vi "Read_Selected_channels.vi"(0 "Filename":path, 1 "Valid Channel Options":string[][](array[string]), 2 "Template Names":string[](array[string]), 3 "Data string":string, 5 "All Channels Present":string[](array[string]), 6 "End Of File already Reached?":bool, 9 "Start of data (bytes)":i32, 12 "Filetype":string, 14 "Ignore When":string[][](array[string])) -> (4 "Non-Blank Rows":i32[](array[numeric]), 8 "Deleted Rows":string[][](array[string]), 10 "Output Values":string[][](array[string]))   [LabVIEW 2015]
uses:
  Data_plotting_vis/Results_plotter_Global.vi
panel:
  out "Case":string
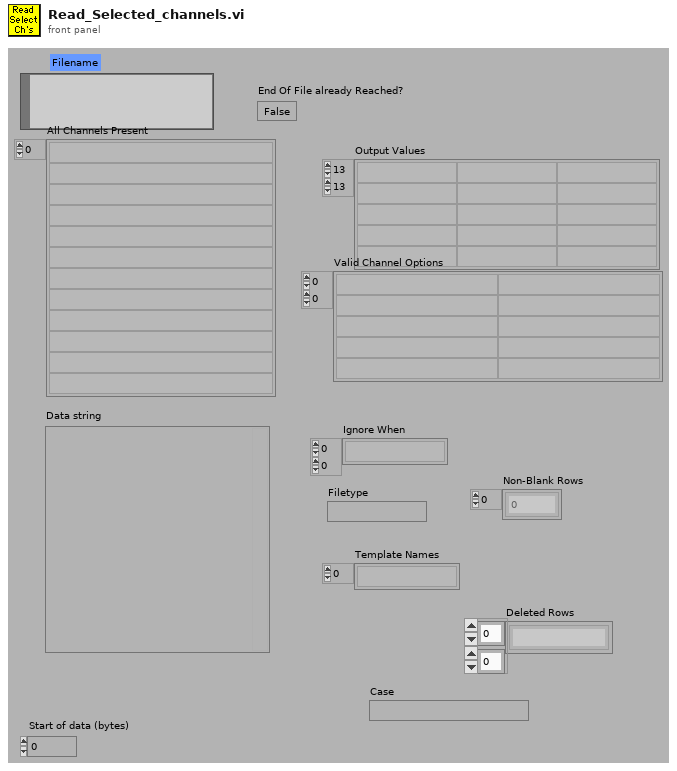
[diagram p1: front panel]
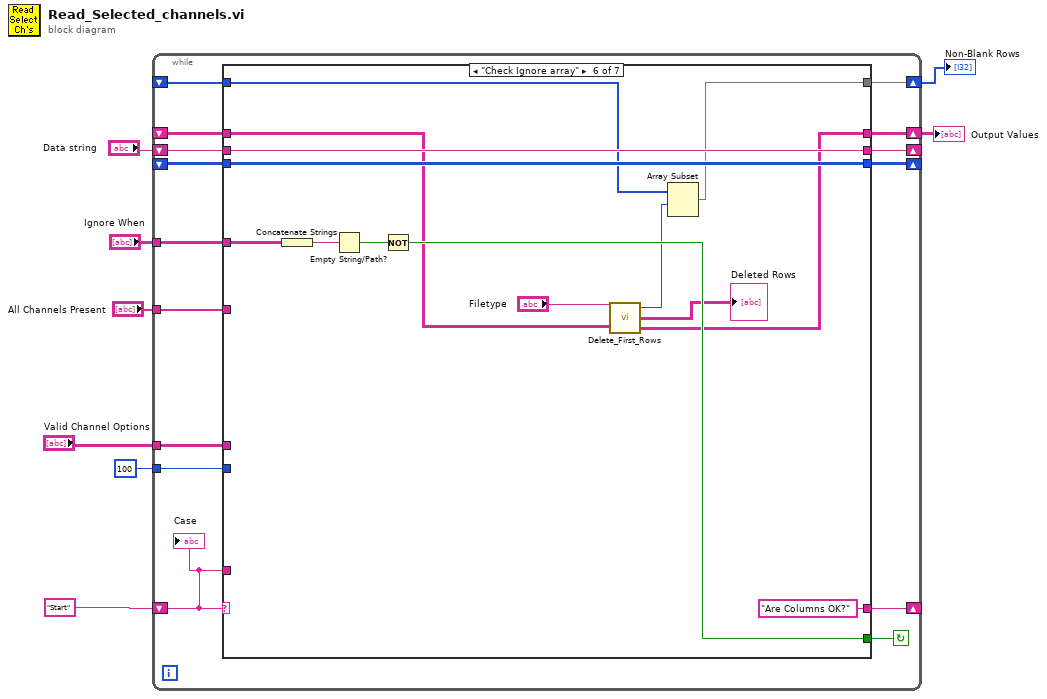
[diagram p0: block diagram]
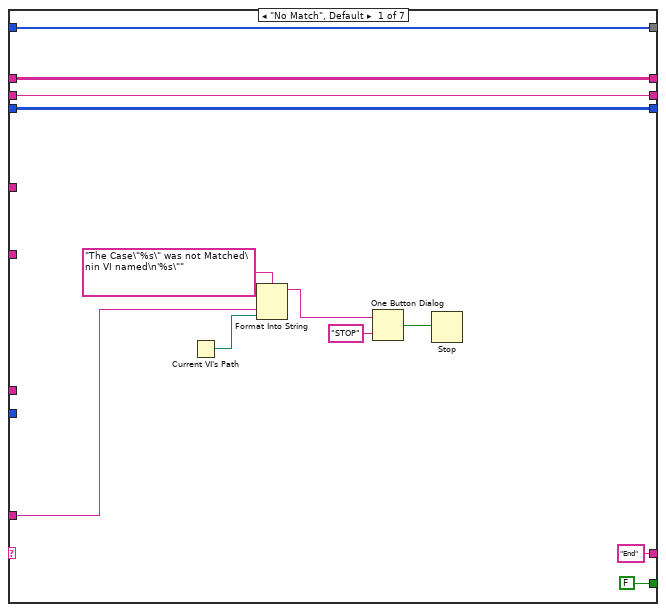
[diagram p2: hidden frame]
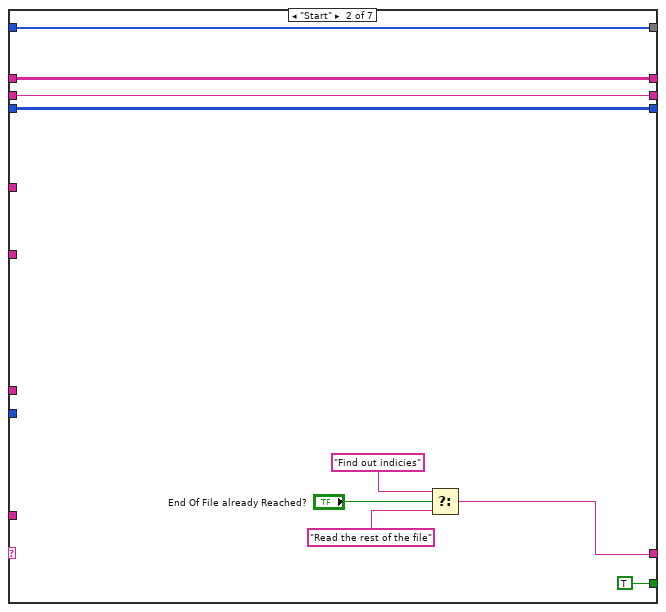
[diagram p3: hidden frame]
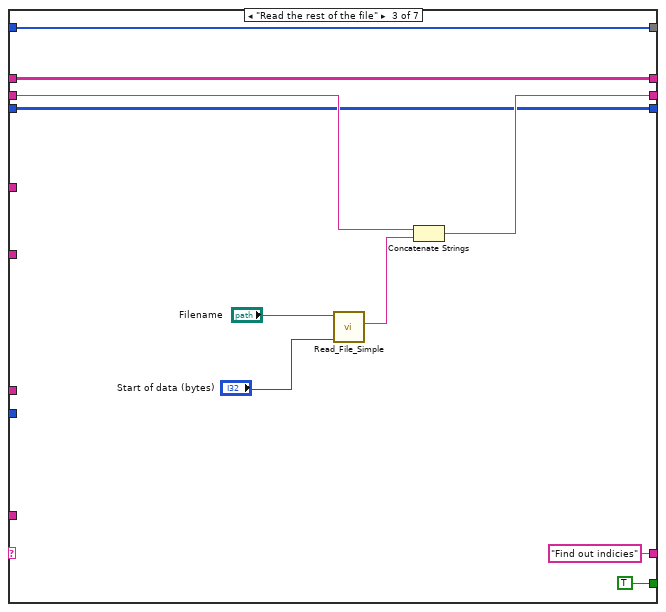
[diagram p4: hidden frame]
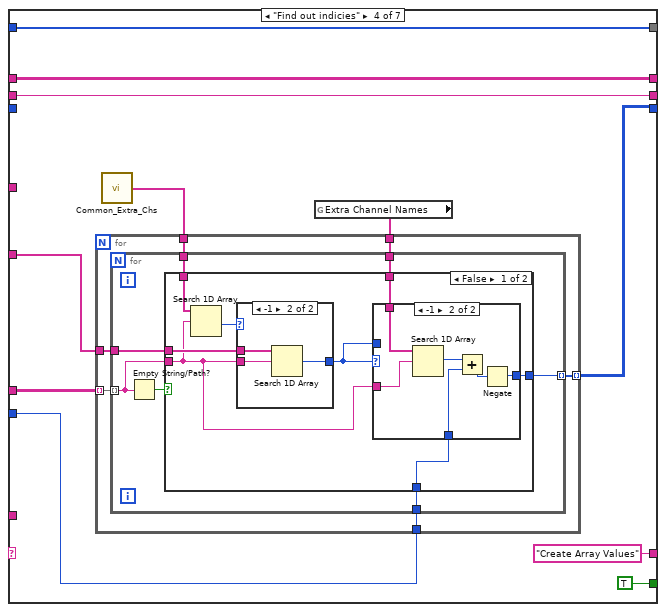
[diagram p5: hidden frame]
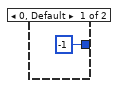
[diagram p6: hidden frame]
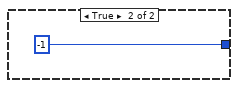
[diagram p8: hidden frame]
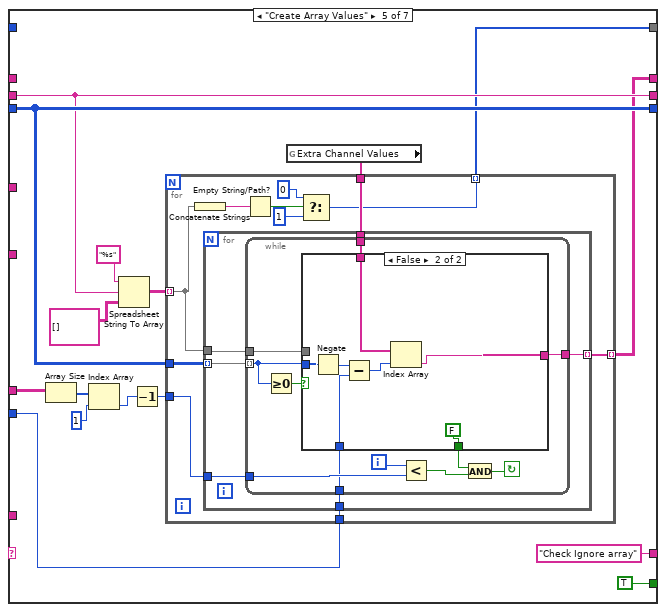
[diagram p9: hidden frame]
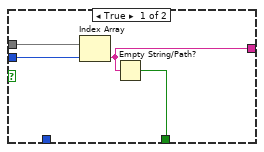
[diagram p10: hidden frame]
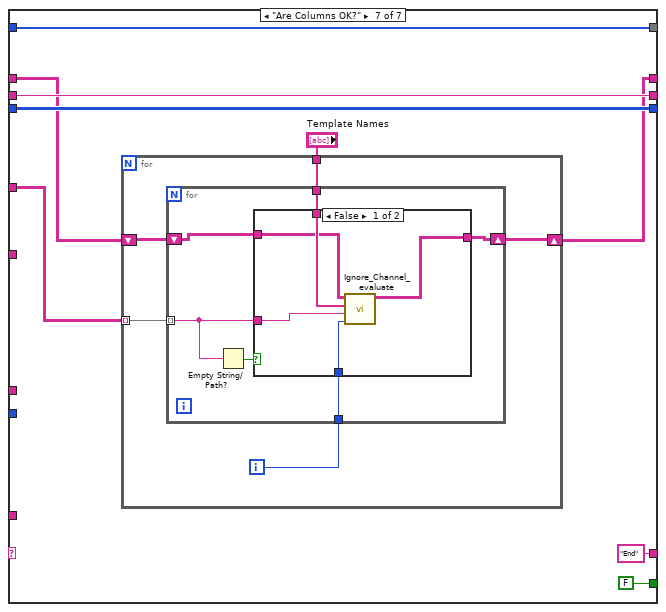
[diagram p11: hidden frame]
diagram:
  n1 = while {
    tunnel: "Ignore When" -> [w11]
    shift-left: _ -> [w12]
    shift-right: [w13] -> w3
    tunnel: 100 ("y") -> [w14]
    tunnel: "Valid Channel Options" -> [w15]
    tunnel: "All Channels Present" -> [w16]
    shift-left: "Data string" -> [w18]
    shift-right: [w17] -> _
    shift-left: _ -> [w20]
    shift-right: [w19] -> _
    shift-left: "Start" -> [w22]
    shift-right: [w21] -> _
    shift-right: [w10] -> w1
    shift-left: _ -> [w9]
    stop <- w23 continue-if-true
    n2 = case shown="\"Check Ignore array\"" w22 {
      tunnel: [FALSE ("Results File?") TRUE ("Results File?") TRUE ("Results File?") TRUE ("Results File?") TRUE ("Results File?") w161 FALSE ("Results File?")] -> w23
      tunnel: w22 -> [w30 _ _ _ _ _ _]
      tunnel: ["End" w39 "Find out indicies" ("f") "Create Array Values" ("f") "Check Ignore array" ("f") "Are Columns OK?" "End"] -> w21
      tunnel: w20 -> [w27 w38 w48 _ w105 w166 w175]
      tunnel: [w27 w38 w48 w59 w105 w166 w175] -> w19
      tunnel: w18 -> [w26 w43 w49 w65 w101 w165 w174]
      tunnel: [w26 w43 w50 w65 w101 w165 w174] -> w17
      tunnel: w16 -> [_ _ _ w60 _ _ _]
      tunnel: w15 -> [_ _ _ w62 w107 _ _]
      tunnel: w14 -> [_ _ _ w58 w111 _ _]
      tunnel: [w25 w37 w46 w57 w100 w159 w168] -> w13
      tunnel: w12 -> [w25 w37 w46 w57 _ w158 w169]
      tunnel: w11 -> [_ _ _ _ _ w164 w172]
      tunnel: [w24 w36 w45 w56 w99 w155 w170] -> w10
      tunnel: w9 -> [w24 w36 w45 w56 _ w156 w170]
      frame "No Match", Default {
        n3 = Current VI's Path() -> (path=w31:path)
        n4 = Format Into String(format string="The Case\"%s\" was not Matched\nin VI named\n'%s\"" ("Format String"), w30, w31) -> (resulting string=w34:string)  [unwired: 2 in, 1 out]
        n5 = One Button Dialog(message=w34, button name ("OK")="STOP") -> (true=w32:bool)
        n6 = Stop(stop? (T)=w32) -> ()
      }
      frame "Start" {
        n7 = Select(t="Find out indicies" ("f"), s="End Of File already Reached?", f="Read the rest of the file") -> (s? t:f=w39:string)
      }
      frame "Read the rest of the file" {
        n8 = call "Read_File_Simple.vi"("Filename"="Filename", "pos offset (bytes:0)"="Start of data (bytes)") -> ("string"=w51:string)  [unwired: 1 in, 7 out]
        n9 = Concatenate Strings(w49, w51) -> (w50:string)
      }
      frame "Find out indicies" {
        n10 = call "Common_Extra_Chs.vi"() -> ("Common Extra Channels"=w55:string[])
        n11 = global read "Results_plotter_Global.vi" "Extra Channel Names"() -> (w61:string[])
        n12 = for {
          tunnel: w60 -> [w71]
          tunnel: w62 -> [w70] mode=indexing
          tunnel: [w69] -> w59 mode=indexing
          tunnel: w58 -> [w68]
          tunnel: w61 -> [w67]
          tunnel: w55 -> [w66]
          n13 = for {
            tunnel: w70 -> [w76] mode=indexing
            tunnel: w71 -> [w78]
            tunnel: [w77] -> w69 mode=indexing
            tunnel: w68 -> [w74]
            tunnel: w67 -> [w73]
            tunnel: w66 -> [w72]
            n14 = Empty String/Path?(string/path=w76) -> (empty?=w75:bool)
            n15 = case shown="False" w75 {
              tunnel: w78 -> [w86 _]
              tunnel: [w85 -1 ("index of element")] -> w77
              tunnel: w76 -> [w80 _]
              tunnel: w74 -> [w83 _]
              tunnel: w73 -> [w82 _]
              tunnel: w72 -> [w81 _]
              frame False {
                n16 = Search 1D Array(1D array=w81, element=w80) -> (index of element=w79:i32)  [unwired: 1 out]
                n17 = case shown="-1" w79 {
                  tunnel: w86 -> [_ w90]
                  tunnel: [-1 ("index of element") w89] -> w84
                  tunnel: w80 -> [_ w88]
                  frame 0, Default {
                  }
                  frame -1 {
                    n18 = Search 1D Array(1D array=w90, element=w88) -> (index of element=w89:i32)  [unwired: 1 out]
                  }
                }
                n19 = case shown="-1" w84 {
                  tunnel: w80 -> [_ w97]
                  tunnel: [w91 w94] -> w85
                  tunnel: w84 -> [w91 _]
                  tunnel: w83 -> [_ w93]
                  tunnel: w82 -> [_ w92]
                  frame 0, Default {
                  }
                  frame -1 {
                    n20 = Search 1D Array(1D array=w92, element=w97) -> (index of element=w96:i32)  [unwired: 1 out]
                    n21 = Add(x=w96, y=w93) -> (x+y=w95:i32)
                    n22 = Negate(x=w95) -> (-x=w94:i32)
                  }
                }
              }
              frame True {
              }
            }
          }
        }
      }
      frame "Create Array Values" {
        n23 = Array Size(array=w107) -> (size(s)=w110:i32[])
        n24 = Index Array(array=w110, index=1 ("Index")) -> (element=w108:i32)
        n25 = Spreadsheet String To Array(format string="%s", spreadsheet string=w101, array type (2D Dbl)=string[][] []) -> (array=w102:string[][])  [unwired: 1 out]
        n26 = Decrement(x=w108) -> (x-1=w106:i32)
        n27 = global read "Results_plotter_Global.vi" "Extra Channel Values"() -> (w112:string[])
        n28 = for {
          tunnel: w105 -> [w125]
          tunnel: w102 -> [w119] mode=indexing
          tunnel: [w124] -> w100 mode=indexing
          tunnel: w111 -> [w123]
          tunnel: w112 -> [w122]
          tunnel: w106 -> [w121]
          tunnel: [w117] -> w99 mode=indexing
          n29 = Concatenate Strings(w119) -> (w120:string)
          n30 = for {
            tunnel: w125 -> [w129] mode=indexing
            tunnel: w119 -> [w131]
            tunnel: [w130] -> w124 mode=indexing
            tunnel: w121 -> [w128]
            tunnel: w123 -> [w127]
            tunnel: w122 -> [w126]
            n31 = while {
              tunnel: w126 -> [w132]
              tunnel: w127 -> [w133]
              tunnel: w128 -> [w139]
              tunnel: w129 -> [w135] mode=indexing
              tunnel: [w141] -> w130
              tunnel: w131 -> [w142]
              i -> [w140]
              stop <- w137 continue-if-true
              n32 = Greater Or Equal To 0?(x=w135) -> (x >= 0?=w134:bool)
              n33 = case shown="False" w134 {
                tunnel: w142 -> [w146 _]
                tunnel: [w144 w153] -> w141
                tunnel: w135 -> [w145 w152]
                tunnel: [w143 FALSE] -> w136
                tunnel: w133 -> [_ w150]
                tunnel: w132 -> [_ w147]
                frame True {
                  n34 = Index Array(array=w146, index=w145) -> (element=w144:string)
                  n35 = Empty String/Path?(string/path=w144) -> (empty?=w143:bool)
                }
                frame False {
                  n36 = Negate(x=w152) -> (-x=w151:i32)
                  n37 = Subtract(x=w151, y=w150) -> (x-y=w149:i32)
                  n38 = Index Array(array=w147, index=w149) -> (element=w153:string)
                }
              }
              n39 = Less?(x=w140, y=w139) -> (x < y?=w138:bool)
              n40 = And(x=w136, y=w138) -> (x .and. y?=w137:bool)
            }
          }
          n41 = Empty String/Path?(string/path=w120) -> (empty?=w118:bool)
          n42 = Select(t=0, s=w118, f=1) -> (s? t:f=w117:i32)
        }
      }
      frame "Check Ignore array" {
        n43 = Concatenate Strings(w164) -> (w163:string)
        n44 = Empty String/Path?(string/path=w163) -> (empty?=w162:bool)
        n45 = Not(x=w162) -> (.not. x?=w161:bool)
        n46 = call "Delete_First_Rows.vi"("File Type"="Filetype", "Data In"=w158) -> ("Rows removed"=w157:i32, "Deleted Rows"=→"Deleted Rows":string[][], "Data Out"=w159:string[][])
        n47 = Array Subset(array=w156, index=w157) -> (w155:i32[])  [unwired: 1 in]
      }
      frame "Are Columns OK?" {
        n48 = for {
          tunnel: "Template Names" -> [w181]
          tunnel: w172 -> [w180] mode=indexing
          shift-right: [w179] -> w168
          shift-left: w169 -> [w178]
          i -> [w177]
          n49 = for {
            tunnel: w181 -> [w187]
            tunnel: w180 -> [w185] mode=indexing
            shift-right: [w184] -> w179
            shift-left: w178 -> [w183]
            tunnel: w177 -> [w182]
            n50 = Empty String/Path?(string/path=w185) -> (empty?=w186:bool)
            n51 = case shown="False" w186 {
              tunnel: w187 -> [w192 _]
              tunnel: w185 -> [w191 _]
              tunnel: [w190 w193] -> w184
              tunnel: w183 -> [w189 w193]
              tunnel: w182 -> [w188 _]
              frame False {
                n52 = call "Ignore_Channel_evaluate.vi"("Column Index"=w188, "Ignore When String"=w191, "Template Names"=w192, "Data"=w189) -> ("Data Out"=w190:string[][])  [unwired: 3 in]
              }
              frame True {
              }
            }
          }
        }
      }
    }
    "Case" <- w22
  }
  "Output Values" <- w3
  "Non-Blank Rows" <- w1
